vi "Enumerate TTLs.vi"(8 "error in (no error)":errorcluster, 11 "State in":refnum<class "State.lvclass">) -> (0 "error out":errorcluster, 2 "TTLs":string[](array[string]), 3 "State out":refnum<class "State.lvclass">)   [LabVIEW 2020, in "State.lvclass"]
uses:
  State.lvclass
  State.lvclass/State.ctl
  Termination/Termination.lvclass/Termination.ctl
  TTL VIs/Control Classes/Base Class/TTLController.lvclass/TTLController.ctl
  Timeout/Timeout.lvclass/Timeout.ctl
  TTL VIs/Control Classes/Base Class/Read Name.vi
  Termination/Read TTL.vi
  Timeout/Read TTL.vi
  TTL VIs/Control Classes/Base Class/TTLController.lvclass
  Termination/Termination.lvclass
  Timeout/Timeout.lvclass
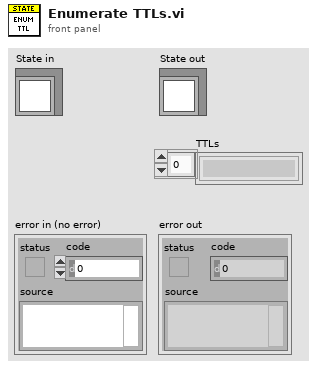
[diagram p1: front panel]
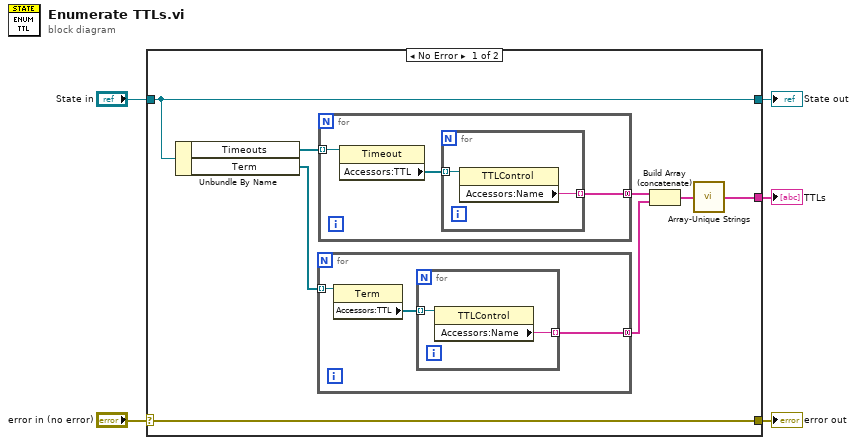
[diagram p0: block diagram]
diagram:
  n1 = case shown="No Error" "error in (no error)" {
    selector: "error in (no error)" -> [w13 w25]
    tunnel: [w13 w25] -> w4
    tunnel: [w12 w24] -> w2
    tunnel: "State in" -> [w12 w24]
    tunnel: [w6 _] -> w1
    frame No Error {
      n2 = Unbundle By Name(w12) -> ("Timeouts"=w11:refnum<class "Timeout.lvclass">[], "Term"=w10:refnum<class "Termination.lvclass">[])
      n3 = for {
        tunnel: w10 -> [w15] mode=indexing
        tunnel: [w14] -> w8 mode=concatenating
        n4 = property class="Term"(reference=w15) -> ("Accessors:TTL"=w16:refnum<class "TTLController.lvclass">[])  [unwired: 1 in, 2 out]
        n5 = for {
          tunnel: w16 -> [w18] mode=indexing
          tunnel: [w17] -> w14 mode=indexing
          n6 = property class="TTLControl"(reference=w18) -> ("Accessors:Name"=w17:string)  [unwired: 1 in, 2 out]
        }
      }
      n7 = for {
        tunnel: w11 -> [w21] mode=indexing
        tunnel: [w19] -> w9 mode=concatenating
        n8 = property class="Timeout"(reference=w21) -> ("Accessors:TTL"=w20:refnum<class "TTLController.lvclass">[])  [unwired: 1 in, 2 out]
        n9 = for {
          tunnel: w20 -> [w23] mode=indexing
          tunnel: [w22] -> w19 mode=indexing
          n10 = property class="TTLControl"(reference=w23) -> ("Accessors:Name"=w22:string)  [unwired: 1 in, 2 out]
        }
      }
      n11 = Build Array (concatenate)(w9, w8) -> (w7:string[])
      n12 = call "Array-Unique Strings.vi"("Strings"=w7) -> ("Unique strings"=w6:string[])  [unwired: 4 in]
    }
    frame Error {
    }
  }
  "error out" <- w4
  "State out" <- w2
  "TTLs" <- w1
